vi "array_to_table_SubVI).vi"(11 "Array in":dbl[][](array[numeric])) -> (3 "Array out":string[][](array[string]))   [LabVIEW 2022 SP3]
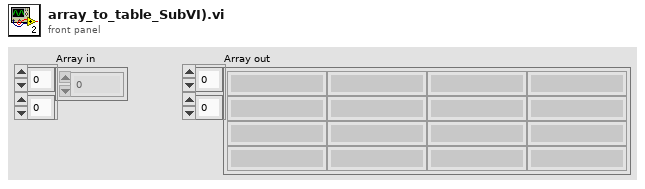
[diagram p1: front panel]
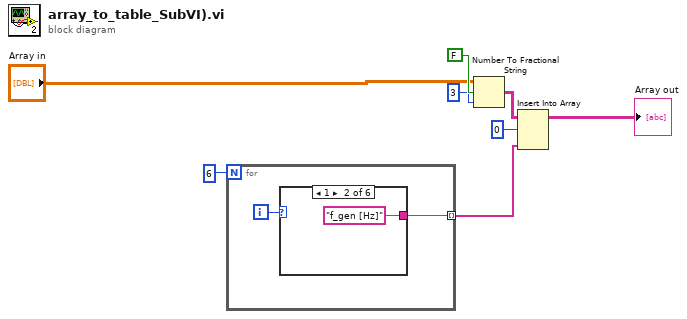
[diagram p0: block diagram]
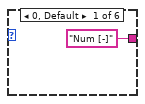
[diagram p2: hidden frame]
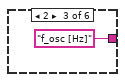
[diagram p3: hidden frame]
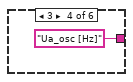
[diagram p4: hidden frame]
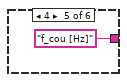
[diagram p5: hidden frame]
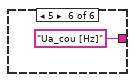
[diagram p6: hidden frame]
diagram:
  n1 = for {
    N: 6 -> [_]
    tunnel: [w9] -> w6 mode=indexing
    i -> [w10]
    n2 = case shown="1" w10 {
      tunnel: ["Num [-]" "f_gen [Hz]" "f_osc [Hz]" "Ua_osc [Hz]" "f_cou [Hz]" "Ua_cou [Hz]"] -> w9
      frame 0, Default {
      }
      frame 1 {
      }
      frame 2 {
      }
      frame 3 {
      }
      frame 4 {
      }
      frame 5 {
      }
    }
  }
  n3 = Number To Fractional String(use system decimal point (T)=FALSE, number="Array in", precision (6)=i16 3) -> (F-format string=w5:string[][])  [unwired: 1 in]
  n4 = Insert Into Array(array=w5, index (row)=0, new element=w6) -> (→"Array out":string[][])  [unwired: 1 in]
